vi "OnbuttonDown.vi"(1 "Input":bool) -> (0 "OnButtonDown":bool)   [LabVIEW 2013]
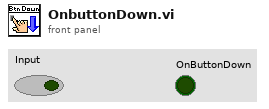
[diagram p1: front panel]
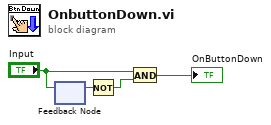
[diagram p0: block diagram]
diagram:
  n1 = feedback #1() -> (w4:bool)  [unwired: 1 in]
  n2 = feedback-in #1("Input") -> ()
  n3 = Not(x=w4) -> (.not. x?=w2:bool)
  n4 = And(x="Input", y=w2) -> (x .and. y?=→"OnButtonDown":bool)
